vi "Handle Last Ack Core.vi"(8 "error in (no error)":errorcluster, 10 "Last Ack":refnum<class "Last Ack.lvclass">, 11 "Mediated Asynchronous Actor in":refnum<class "Mediated Asynchronous Actor.lvclass">) -> (0 "error out":errorcluster, 3 "Mediated Asynchronous Actor out":refnum<class "Mediated Asynchronous Actor.lvclass">)   [LabVIEW 2016, in "Stream Mediator.lvlib" / "Mediated Asynchronous Actor.lvclass"]
doc: "--\nCopyright © 2017 Composed SystemsI All rights reserved.\n\nAuthor: Jon McBee <jon.mcbee@composed.io>\n\nThis library is provided \"AS IS\" ,WITHOUT WARRANTIES OR\nCONDITIONS OF ANY KIND, either express or implied.\n\nComposed Systems -- composed.io\n\nStream 0.0.1.1\nJon McBee - Composed Systems\nCopyright (c) 2017, Composed Systems"
uses:
  <userlib>/Composed Systems/Stream/Mediator/Classes/Mediated Asynchronous Actor/Mediated Asynchronous Actor.lvclass
  <userlib>/Composed Systems/Stream/Mediator/Classes/Message Command Last Ack/Last Ack.lvclass
  <userlib>/Composed Systems/Stream/Mediator/Classes/Message Command Last Ack/Last Ack.lvclass/Last Ack.ctl
  <userlib>/Composed Systems/Stream/Mediator/Classes/Message Transport Queue/Message Transport Queue.lvclass
  C:/Program Files (x86)/National Instruments/LabVIEW 2016/user.lib/Composed Systems/Stream/Mediator/Classes/Message Transport Interface/Message Transport Interface.lvclass
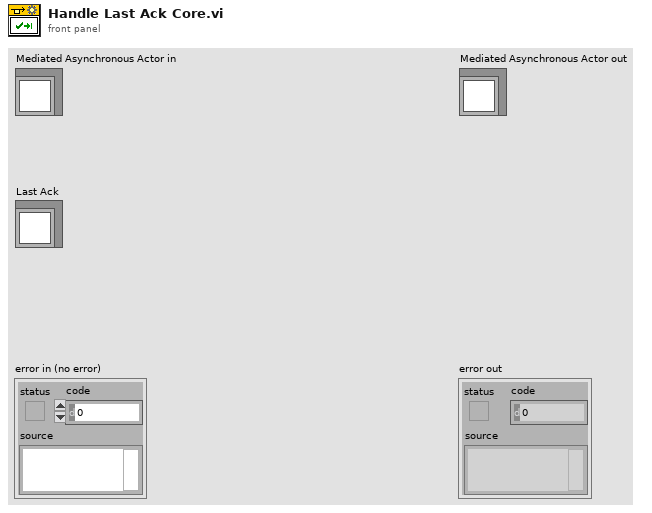
[diagram p1: front panel]
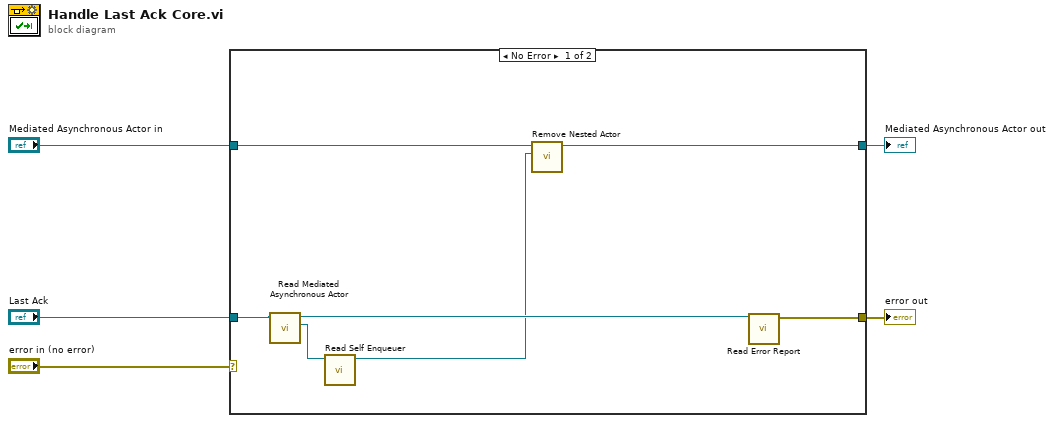
[diagram p0: block diagram]
diagram:
  n1 = case shown="No Error" "error in (no error)" {
    selector: "error in (no error)" -> [_ w14]
    tunnel: [w12 w14] -> w4
    tunnel: [w7 w13] -> w2
    tunnel: "Mediated Asynchronous Actor in" -> [w11 w13]
    tunnel: "Last Ack" -> [w10 _]
    frame No Error {
      n2 = call <userlib>:"Read Mediated Asynchronous Actor.vi"("Last Ack in"=w10) -> ("Stream Mediator.lvlib:Mediated Asynchronous Actor.lvclass"=w8:refnum<class "Mediated Asynchronous Actor.lvclass">, "Last Ack out"=w9:refnum<class "Last Ack.lvclass">)  [unwired: 9 in]
      n3 = call <userlib>:"Read Self Enqueuer.vi"("Mediated Asynchronous Actor in"=w8) -> ("Self Enqueuer"=w6:refnum<class "Message Transport Queue.lvclass">)  [unwired: 10 in]
      n4 = call <userlib>:"Remove Nested Actor.vi"("Nested Mediated Asynchronous Actor's Message Transport"=w6, "Mediated Asynchronous Actor in"=w11) -> ("Mediated Asynchronous Actor out"=w7:refnum<class "Mediated Asynchronous Actor.lvclass">)  [unwired: 8 in, 1 out]
      n5 = call <userlib>:"Read Error Report.vi"("Last Ack in"=w9) -> ("Error Report"=w12:errorcluster)  [unwired: 9 in, 1 out]
    }
    frame Error {
    }
  }
  "error out" <- w4
  "Mediated Asynchronous Actor out" <- w2
